vi "Excel表格读.vi"(9 "单页表名称":string="接触面", 11 "路径":path=path "E:/广东华旃/广东华旃864插座位置度CCD检测-all/广东华旃插座位置度CCD检测-20200721/接触面PIN 正位度-864 设备调试比对-3号样品-7.16.xlsx") -> (2 "Excel表格原始数据":string[][](array[string]))   [LabVIEW 2014]
uses:
  <vilib>/Utility/file.llb/Read From Spreadsheet File (string).vi
  <vilib>/Utility/NIReport.llb/NI_report.lvclass
  <vilib>/Utility/NIReport.llb/Excel/NI_Excel.lvclass
  <vilib>/addons/_office/NI_ReportGenerationToolkit.lvlib
  <vilib>/addons/_office/excel.llb/Excel Get Data ([str]).vi
panel:
  out "all rows":string[][](array[string]) caption="所有行"
  out "数值":i32
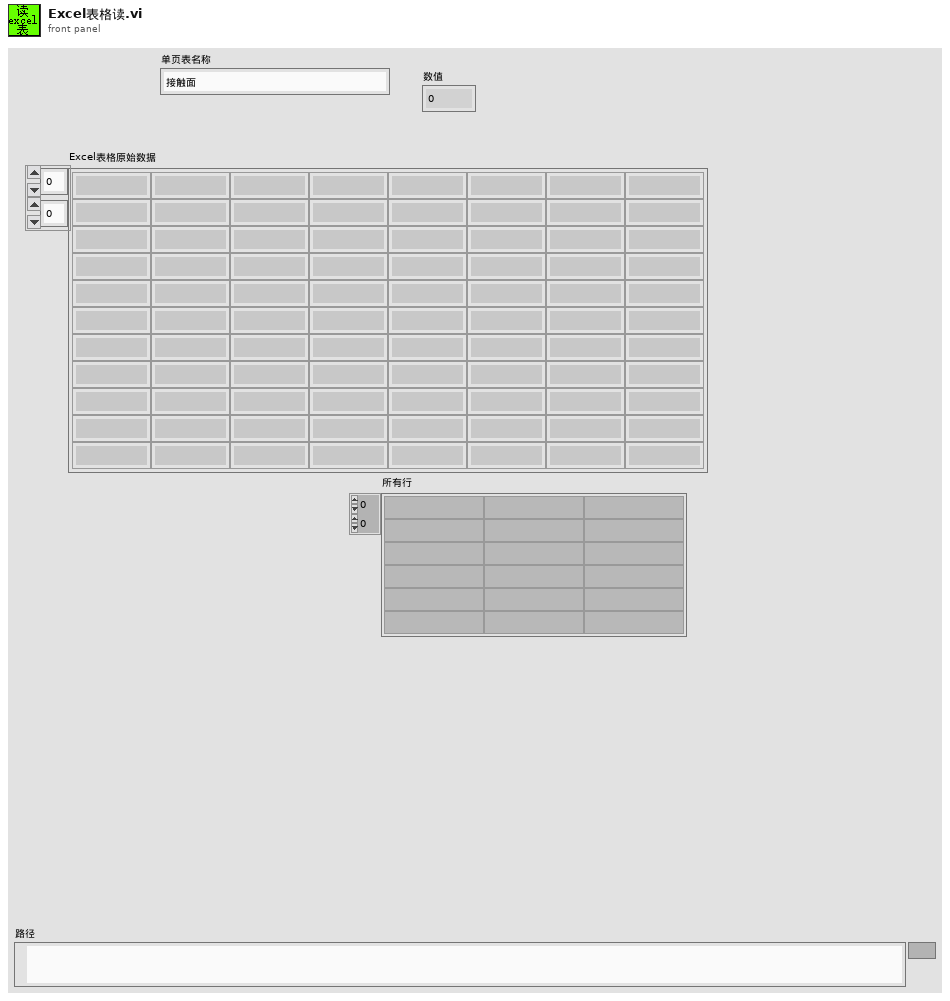
[diagram p1: front panel]
types:
  T1 = enum16{"maximized", "minimized", "normal", "no change"}
  T2 = enum16{"Standard Report", "HTML", "Word", "Excel"}
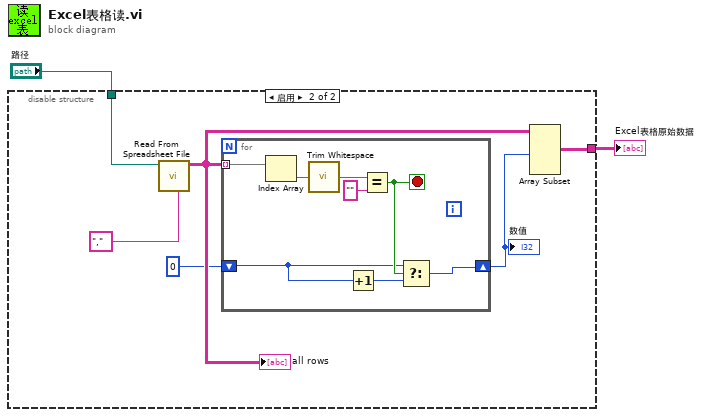
[diagram p0: block diagram]
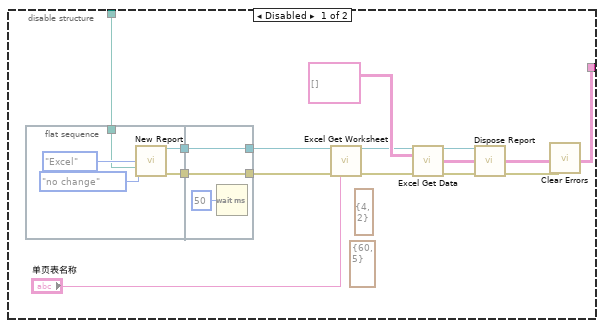
[diagram p2: hidden frame]
diagram:
  n1 = disable-structure shown="启用" {
    disable-tunnel: "路径" -> [w13 w29]
    disable-tunnel: [w4 w26] -> w1
    frame Disabled {
      (unwired) cluster{"row":i32, "column":i32} {"row"=60, "column"=5} ("end (-1, -1)")
      (unwired) cluster{"row":i32, "column":i32} {"row"=4, "column"=2} ("start (-1, -1)")
      n2 = flat-sequence {
        tunnel: [w20] -> w15
        tunnel: w13 -> [w17]
        tunnel: [w16] -> w14
        tunnel: [w23] -> w9
        tunnel: w15 -> [w23]
        tunnel: [w21] -> w8
        tunnel: w14 -> [w21]
        frame #0 {
          n3 = call <vilib>:"New Report.vi"("window state (normal)"=T1."no change", "report type"=T2."Excel", "template (empty)"=w17) -> ("report out"=w20:refnum<class "NI_report.lvclass">, "error out"=w16:errorcluster)  [unwired: 11 in]
        }
        frame #1 {
          n4 = Wait (ms)(milliseconds to wait=u32 50 ("等待时间（毫秒）")) -> ()  [unwired: 1 out]
        }
      }
      n5 = call <vilib>:"Excel Get Worksheet.vi"("report in"=w9, "error in (no error)"=w8, "name (\"\")"="单页表名称") -> ("report out"=w11:refnum<class "NI_report.lvclass">, "error out"=w10:errorcluster)  [unwired: 11 in]
      n6 = call-poly <vilib>:"Excel Get Data.vi"("report in"=w11, "data type"=string[][] [], "error in (no error)"=w10) -> ("report out"=w3:refnum<class "NI_report.lvclass">, "data"=w4:string[][], "error out"=w5:errorcluster)  [unwired: 10 in]
      n7 = call-dynamic "Dispose Report.vi"("report in"=w3, "error in (no error)"=w5) -> ("error out"=w6:errorcluster)  [unwired: 13 in]
      n8 = call <vilib>:"Clear Errors.vi"("error in (no error)"=w6) -> ()  [unwired: 5 in, 2 out]
    }
    frame Enabled {
      n9 = call-poly <vilib>:"Read From Spreadsheet File.vi"("delimiter (\\t)"="," ("delimiter (\\t)"), "file path (dialog if empty)"=w29) -> ("all rows"=w27:string[][])  [unwired: 5 in, 4 out]
      "all rows" <- w27
      n10 = for {
        tunnel: w27 -> [w37] mode=indexing
        shift-right: [w31] -> w24
        shift-left: 0 -> [w30]
        stop <- w33 stop-if-true
        n11 = Index Array(array=w37) -> (element=w34:string)  [unwired: 1 in]
        n12 = call <vilib>:"Trim Whitespace.vi"("string"=w34) -> ("trimmed string"=w36:string)  [unwired: 1 in]
        n13 = Increment(x=w30) -> (x+1=w32:i32)
        n14 = Equal?(x=w36, y="" ("String")) -> (x = y?=w33:bool)
        n15 = Select(t=w30, s=w33, f=w32) -> (s? t:f=w31:i32)
      }
      "数值" <- w24
      n16 = Array Subset(array=w27, length (row)=w24) -> (w26:string[][])  [unwired: 3 in]
    }
  }
  "Excel表格原始数据" <- w1
